vi "GetLvClassRef.vi"(0 "ClassReaderNative in":refnum<class "ClassReaderNative.lvclass">, 5 "error in (no error)":errorcluster) -> (14 "ClassReaderNative out":refnum<class "ClassReaderNative.lvclass">, 16 "LvClassRef":refnum<vi>, 19 "error out":errorcluster)   [LabVIEW 2020, in "ClassReaderNative.lvclass"]
uses:
  ClassReaderNative.lvclass
  ClassReaderNative.lvclass/ClassReaderNative.ctl
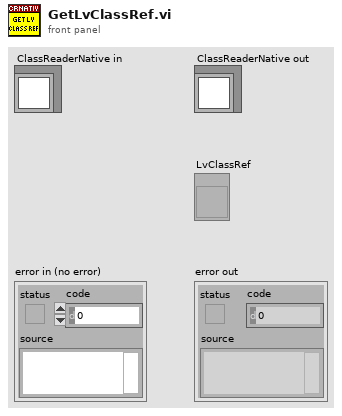
[diagram p1: front panel]
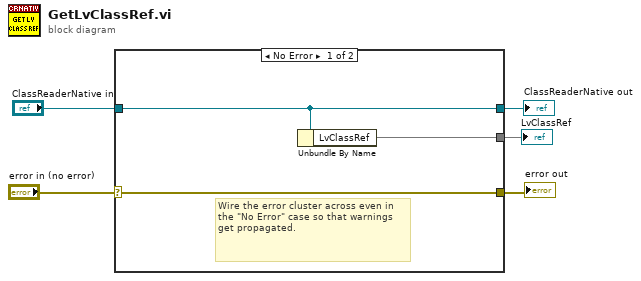
[diagram p0: block diagram]
diagram:
  n1 = case shown="No Error" "error in (no error)" {
    selector: "error in (no error)" -> [w6 w10]
    tunnel: [w6 w10] -> w4
    tunnel: [w8 w9] -> w2
    tunnel: "ClassReaderNative in" -> [w8 w9]
    tunnel: [w7 _] -> w1
    frame No Error {
      # "Wire the error cluster across even in the \"No Error\" case so that warnings get propagated."
      n2 = Unbundle By Name(w8) -> ("LvClassRef"=w7)
    }
    frame Error {
    }
  }
  "error out" <- w4
  "ClassReaderNative out" <- w2
  "LvClassRef" <- w1
